vi "CAL-Speaker Cal Path.vi"(0 "Speaker":T1, 5 "Data Folder":path, 11 "error in (no error)":errorcluster) -> (6 "Cal Path":path, 15 "error out":errorcluster)   [LabVIEW 2020]
uses:
  epl-vi-lib/Utility VIs/Type Defs/Speaker ring.ctl
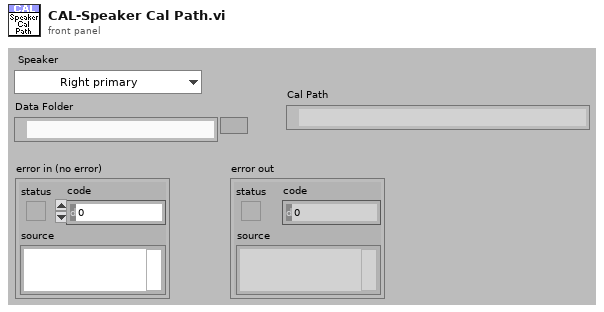
[diagram p1: front panel]
types:
  T1 = typedef "Speaker ring.ctl" = enum16{"Right primary", "Right secondary", "Left primary", "Left secondary"}
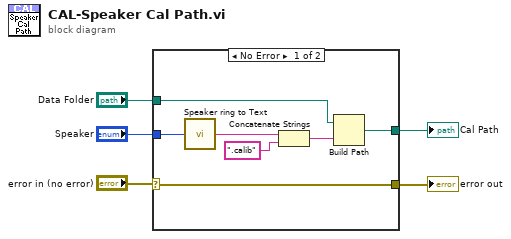
[diagram p0: block diagram]
diagram:
  n1 = case shown="No Error" "error in (no error)" {
    selector: "error in (no error)" -> [w8 w13]
    tunnel: "Speaker" -> [w7 _]
    tunnel: "Data Folder" -> [w11 _]
    tunnel: [w9 _] -> w2
    tunnel: [w8 w13] -> w1
    frame No Error {
      n2 = call "Speaker ring to Text.vi"("Speaker"=w7) -> ("Text"=w6:string)
      n3 = Concatenate Strings(w6, ".calib" ("string")) -> (w10:string)
      n4 = Build Path(base path=w11, name or relative path=w10) -> (appended path=w9:path)
    }
    frame Error {
    }
  }
  "error out" <- w1
  "Cal Path" <- w2
